vi "SetTarget.vi"(8 "error in":errorcluster, 9 "Position":u16, 10 "Channel":u8, 11 "VISA resource name":refnum<visa-resource-name>) -> (0 "error out":errorcluster, 3 "VISA resource name out":refnum<visa-resource-name>)   [LabVIEW 2023, in "Maestro.lvlib"]
uses:
  Maestro.lvlib
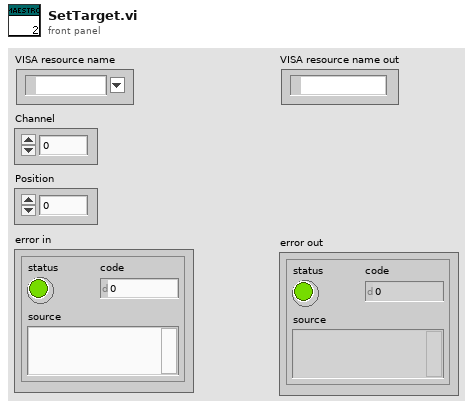
[diagram p1: front panel]
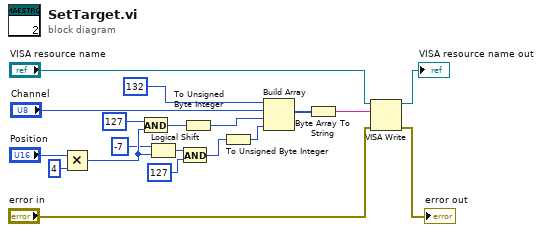
[diagram p0: block diagram]
diagram:
  n1 = Multiply(x="Position", y=u16 4) -> (x*y=w9:u16)
  n2 = And(x=u8 127, y=w9) -> (x .and. y?=w13:u16)
  n3 = Logical Shift(y=i16 -7, x=w9) -> (x << y=w10:u16)
  n4 = And(x=w10, y=u8 127) -> (x .and. y?=w11:u16)
  n5 = To Unsigned Byte Integer(number=w13) -> (unsigned 8bit integer=w14:u8)
  n6 = To Unsigned Byte Integer(number=w11) -> (unsigned 8bit integer=w12:u8)
  n7 = Build Array(u8 132, "Channel", w14, w12) -> (w6:u8[])
  n8 = Byte Array To String(unsigned byte array=w6) -> (string=w5:string)
  n9 = VISA Write(VISA resource name="VISA resource name", write buffer=w5, error in (no error)="error in") -> (VISA resource name out=→"VISA resource name out":refnum<visa-resource-name>, error out=→"error out":errorcluster)  [unwired: 1 out]
